vi "_Delete Tables Module.vi"(6 "connection information":path, 8 "error in (no error)":errorcluster, 11 "Mode (Get Connection)":T2=enum."Get Connection") -> (0 "error out":errorcluster, 3 "connection reference":T1)   [LabVIEW 2013]
doc: "Wrapper for database module. Low level module is reentrant, this wrapper creates an instance for the scanner code.s"
uses:
  DB Connection Mode enum.ctl
  Utility/database/Connection.llb/Conn ObjectReference.ctl
  Database Lib.lvlib
  Utility/database/NI_Database_API_64.lvlib
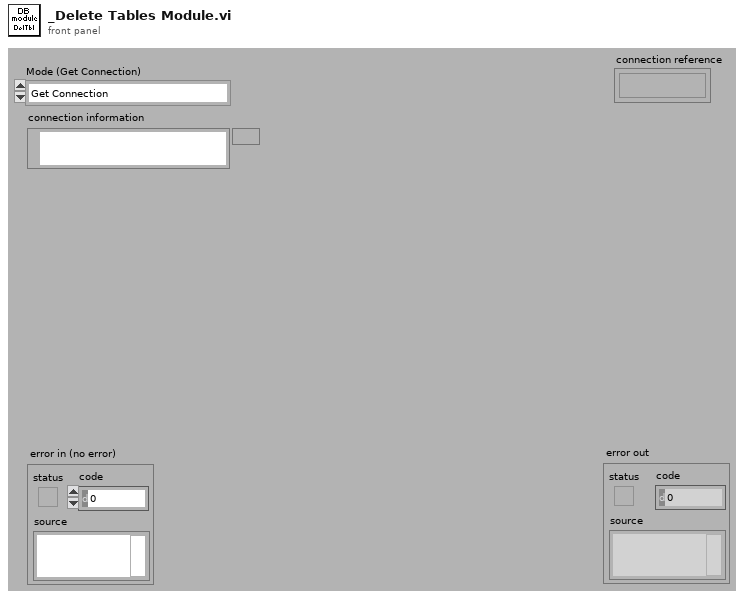
[diagram p1: front panel]
types:
  T1 = typedef "NI_Database_API_64.lvlib/Conn ObjectReference.ctl" = refnum<k1>
  T2 = typedef "Database Lib.lvlib/DB Connection Mode enum.ctl" = enum16{"Connect", "Get Connection", "Disconnect"}
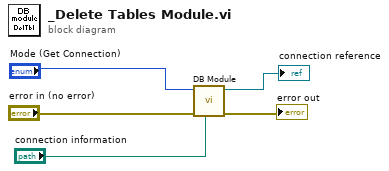
[diagram p0: block diagram]
diagram:
  n1 = call "DB Module.vi"("connection information"="connection information", "error in (no error)"="error in (no error)", "Mode (Get Connection)"="Mode (Get Connection)") -> ("error out"=→"error out":errorcluster, "connection reference"=→"connection reference":T1)  [unwired: 7 out]
